vi "AddCredit.vi"(8 "error in (no error)":errorcluster, 10 "Credit Added":dbl, 11 "Messages Actor in":refnum<class "Messages Actor.lvclass">) -> (0 "error out":errorcluster, 3 "Messages Actor out":refnum<class "Messages Actor.lvclass">)   [LabVIEW 2020, in "Messages Actor.lvlib" / "Messages Actor.lvclass"]
uses:
  Messages Actor.lvclass
  Messages Actor.lvclass/Messages Actor.ctl
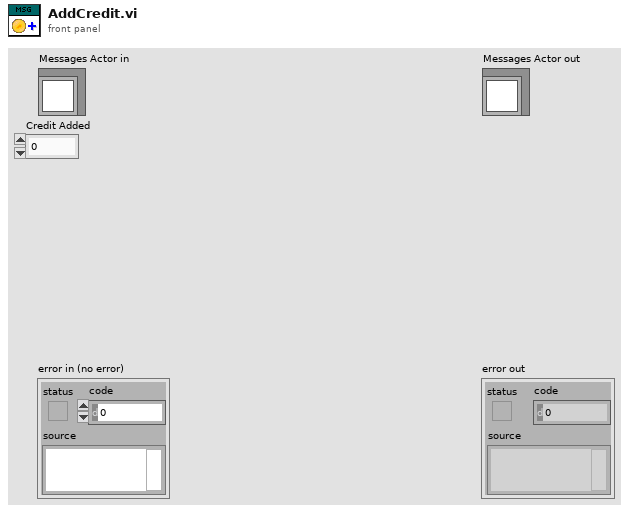
[diagram p1: front panel]
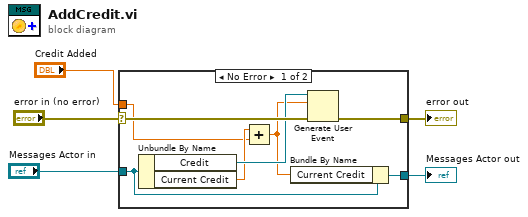
[diagram p0: block diagram]
diagram:
  n1 = case shown="No Error" "error in (no error)" {
    selector: "error in (no error)" -> [w13 w15]
    tunnel: [w11 w15] -> w4
    tunnel: [w7 w14] -> w2
    tunnel: "Messages Actor in" -> [w12 w14]
    tunnel: "Credit Added" -> [w8 _]
    frame No Error {
      n2 = Unbundle By Name(w12) -> ("Credit"=w10:refnum<user-event>, "Current Credit"=w9:dbl)
      n3 = Add(x=w9, y=w8) -> (x+y=w6:dbl)
      n4 = Bundle By Name(cluster=w12, "Current Credit"=w6) -> (w7:refnum<class "Messages Actor.lvclass">)
      n5 = Generate User Event(user event=w10, event data cluster=w6, error in=w13) -> (error out=w11:errorcluster)  [unwired: 1 in, 1 out]
    }
    frame Error {
    }
  }
  "error out" <- w4
  "Messages Actor out" <- w2
